vi "Write Trigger Source.vi"(8 "error in (no error)":errorcluster, 10 "Trigger Source":string, 11 "Camera in":refnum<class "Camera.lvclass">) -> (0 "error out":errorcluster, 3 "Camera":refnum<class "Camera.lvclass">)   [LabVIEW 2020, in "Camera.lvclass"]
uses:
  Camera.lvclass
  Camera.lvclass/Camera.ctl
  Value Set Action.ctl
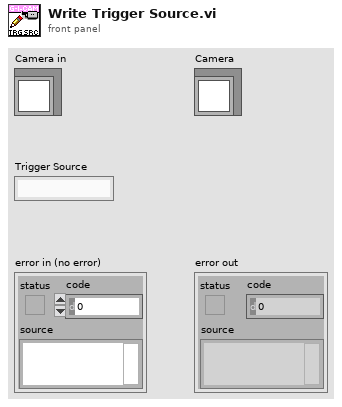
[diagram p1: front panel]
types:
  T1 = typedef "Camera.lvclass/Value Set Action.ctl" = enum16{"Set and Validate", "Set Only"}
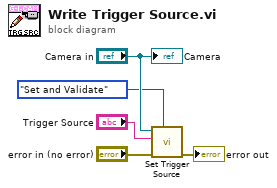
[diagram p0: block diagram]
diagram:
  n1 = call "Set Trigger Source.vi"("Action (Default: Set and Validate)"=Value_Set_Action."Set and Validate", "error in (no error)"="error in (no error)", "Source"="Trigger Source", "Camera in"="Camera in") -> ("error out"=→"error out":errorcluster)  [unwired: 6 in, 1 out]
  "Camera" <- "Camera in"
